vi "client example - sine wave - analog.vi"() -> ()   [LabVIEW 2021]
uses:
  controls/generation status.ctl
  controls/sine wave properties.ctl
  controls/analog output settings.ctl
  controls/terminal configuration.ctl
  AudioGeneration/Configure - Analog.vi
  AudioGeneration/AudioGeneration.lvclass
  controls/AudioGenTypeDefs.lvlib
panel:
  in  "sine wave properties":T1=[{"frequency"=1000.0, "amplitude"=1.0, "phase"=0.0}, {"frequency"=1000.0, "amplitude"=2.0, "phase"=30.0}]
  in  "update":bool
  in  "terminal configuration":i32(ring)=10106 items=["Default"=-1, "RSE"=10083, "Differential"=10106, "Pseudodifferential"=12529]
  in  "range":dbl=5.0
  in  "DAQmx Physical Channel":tag="PXI1Slot4/ao0:1"
  out "status":T2
  in  "stop":bool
  out "error out":errorcluster
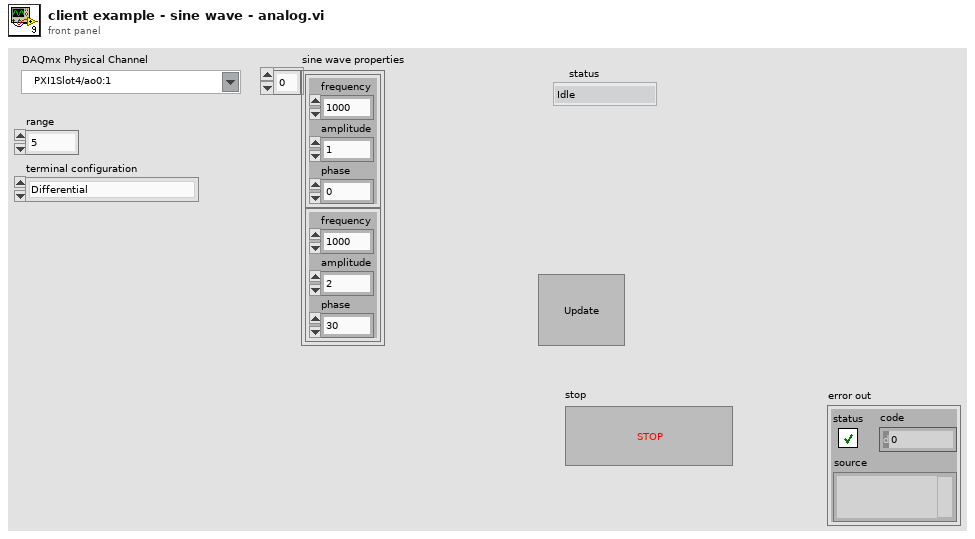
[diagram p1: front panel]
types:
  T1 = typedef "AudioGenTypeDefs.lvlib/sine wave properties.ctl" = cluster{"frequency":dbl, "amplitude":dbl, "phase":dbl}[]
  T2 = typedef "AudioGenTypeDefs.lvlib/generation status.ctl" = enum16{"Idle", "Committed", "Active"}
  T3 = typedef "AudioGenTypeDefs.lvlib/analog output settings.ctl" = cluster{"output rate":dbl, "range":dbl, "terminal configuration":T4, "output impedance":dbl, "common mode offset":dbl, "pure tone mode":bool}
  T4 = typedef "AudioGenTypeDefs.lvlib/terminal configuration.ctl" = enum32{"Default", "RSE", "Differential", "Pseudodifferential"}
  T5 = typedef "AudioGenTypeDefs.lvlib/signal settings.ctl" = cluster{"signal type":T6, "properties":string, "output level units":T7}
  T6 = typedef "AudioGenTypeDefs.lvlib/signal type.ctl" = enum16{"Sine", "Dual Tone"}
  T7 = typedef "audio controls.lvlib/digital output level units.ctl" = enum32{"% FS", "dBFS", "V"}
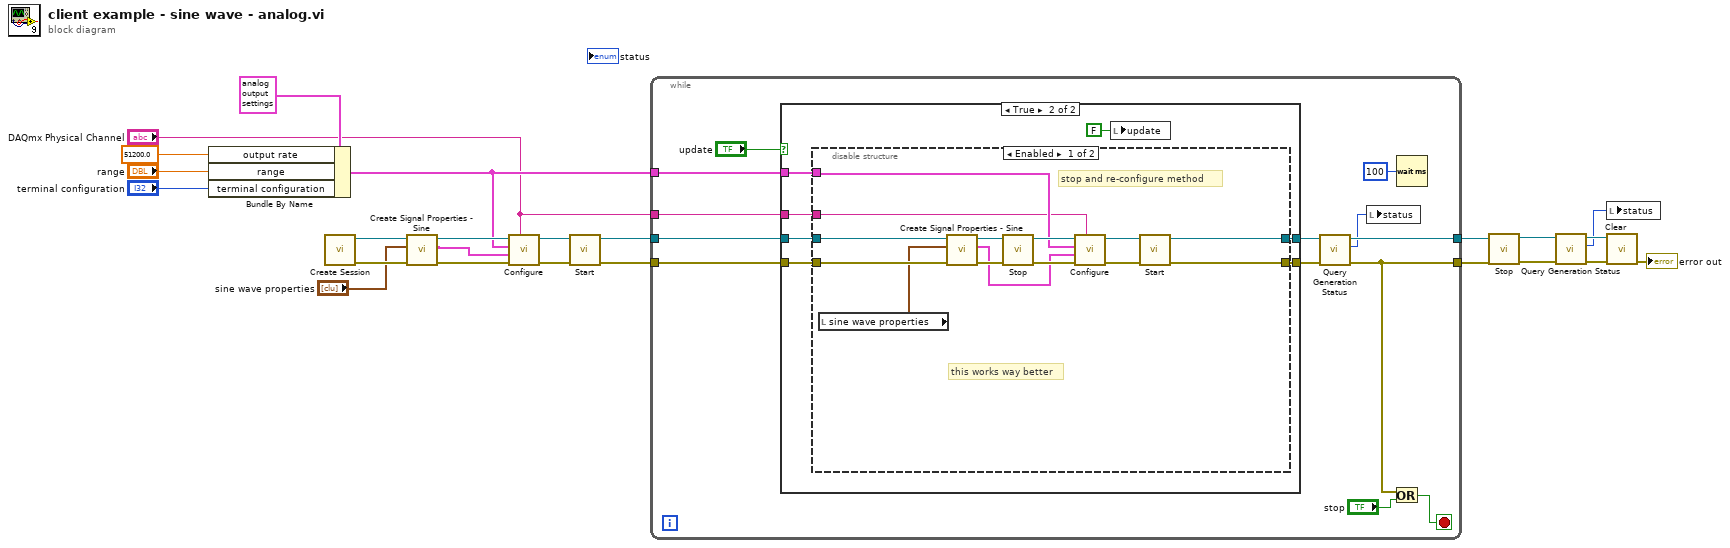
[diagram p0: block diagram]
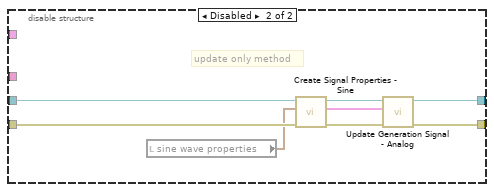
[diagram p3: hidden frame]
diagram:
  n1 = Bundle By Name(cluster=T3 {"output rate"=51200.0, "range"=5.0, "terminal configuration"=enum."Pseudodifferential", "output impedance"=0.0, "common mode offset"=0.0, "pure tone mode"=FALSE} ("output settings"), "output rate"=51200.0 ("output settings.output rate"), "range"="range", "terminal configuration"="terminal configuration") -> (w2:T3)
  n2 = call "Create Session.vi"() -> ("error out"=w9:errorcluster, "session out"=w10:refnum<class "AudioGeneration.lvclass">)  [unwired: 10 in]
  n3 = call "Create Signal Properties - Sine.vi"("error in (no error)"=w9, "sine wave properties"="sine wave properties", "AudioGeneration in"=w10) -> ("error out"=w6:errorcluster, "signal settings"=w7:T5, "AudioGeneration out"=w8:refnum<class "AudioGeneration.lvclass">)  [unwired: 6 in]
  n4 = call-poly "Configure.vi"("DAQmx Physical Channel"="DAQmx Physical Channel", "error in (no error)"=w6, "signal settings"=w7, "output settings"=w2, "AudioGeneration in"=w8) -> ("error out"=w4:errorcluster, "AudioGeneration out"=w5:refnum<class "AudioGeneration.lvclass">)  [unwired: 5 in]
  n5 = call "Start.vi"("error in (no error)"=w4, "AudioGeneration in"=w5) -> ("error out"=w20:errorcluster, "AudioGeneration out"=w21:refnum<class "AudioGeneration.lvclass">)  [unwired: 8 in]
  n6 = while {
    tunnel: [w34] -> w23
    tunnel: [w33] -> w22
    tunnel: w21 -> [w31]
    tunnel: w20 -> [w29]
    tunnel: w2 -> [w26]
    tunnel: "DAQmx Physical Channel" -> [w25]
    stop <- w36 stop-if-true
    n7 = case shown="True" "update" {
      tunnel: w31 -> [w39 w43]
      tunnel: w29 -> [w38 w42]
      tunnel: [w38 w46] -> w28
      tunnel: [w39 w45] -> w27
      tunnel: w26 -> [_ w41]
      tunnel: w25 -> [_ w40]
      frame False {
      }
      frame True {
        n8 = disable-structure shown="Enabled" {
          disable-tunnel: [w48 w68] -> w46
          disable-tunnel: [w49 w67] -> w45
          disable-tunnel: w43 -> [w60 w66]
          disable-tunnel: w42 -> [w59 w65]
          disable-tunnel: w41 -> [w53 _]
          disable-tunnel: w40 -> [w47 _]
          frame Enabled {
            # "this works way better"
            # "stop and re-configure method"
            n9 = local read "sine wave properties"() -> (w58:T1)
            n10 = call "Create Signal Properties - Sine.vi"("error in (no error)"=w59, "sine wave properties"=w58, "AudioGeneration in"=w60) -> ("error out"=w57:errorcluster, "signal settings"=w52:T5, "AudioGeneration out"=w56:refnum<class "AudioGeneration.lvclass">)  [unwired: 6 in]
            n11 = call "Stop.vi"("error in (no error)"=w57, "AudioGeneration in"=w56) -> ("error out"=w55:errorcluster, "AudioGeneration out"=w54:refnum<class "AudioGeneration.lvclass">)  [unwired: 8 in]
            n12 = call-poly "Configure.vi"("DAQmx Physical Channel"=w47, "error in (no error)"=w55, "signal settings"=w52, "output settings"=w53, "AudioGeneration in"=w54) -> ("error out"=w51:errorcluster, "AudioGeneration out"=w50:refnum<class "AudioGeneration.lvclass">)  [unwired: 5 in]
            n13 = call "Start.vi"("error in (no error)"=w51, "AudioGeneration in"=w50) -> ("error out"=w48:errorcluster, "AudioGeneration out"=w49:refnum<class "AudioGeneration.lvclass">)  [unwired: 8 in]
          }
          frame Disabled {
            # "update only method"
            n14 = local read "sine wave properties"() -> (w61:T1)
            n15 = call "Create Signal Properties - Sine.vi"("error in (no error)"=w65, "sine wave properties"=w61, "AudioGeneration in"=w66) -> ("error out"=w63:errorcluster, "signal settings"=w62:T5, "AudioGeneration out"=w64:refnum<class "AudioGeneration.lvclass">)  [unwired: 6 in]
            n16 = call "Update Generation Signal - Analog.vi"("error in (no error)"=w63, "signal settings"=w62, "AudioGeneration in"=w64) -> ("error out"=w68:errorcluster, "AudioGeneration out"=w67:refnum<class "AudioGeneration.lvclass">)  [unwired: 7 in]
          }
        }
        n17 = local write "update"(FALSE ("update")) -> ()
      }
    }
    n18 = call "Query Generation Status.vi"("error in (no error)"=w28, "AudioGeneration in"=w27) -> ("error out"=w33:errorcluster, "status"=w32:T2, "AudioGeneration out"=w34:refnum<class "AudioGeneration.lvclass">)  [unwired: 5 in, 2 out]
    n19 = local write "status"(w32) -> ()
    n20 = Or(x=w33, y="stop") -> (x .or. y?=w36:bool)
    n21 = Wait (ms)(milliseconds to wait=u32 100) -> ()  [unwired: 1 out]
  }
  n22 = call "Stop.vi"("error in (no error)"=w22, "AudioGeneration in"=w23) -> ("error out"=w15:errorcluster, "AudioGeneration out"=w19:refnum<class "AudioGeneration.lvclass">)  [unwired: 8 in]
  n23 = call "Query Generation Status.vi"("error in (no error)"=w15, "AudioGeneration in"=w19) -> ("error out"=w17:errorcluster, "status"=w16:T2, "AudioGeneration out"=w18:refnum<class "AudioGeneration.lvclass">)  [unwired: 5 in, 2 out]
  n24 = local write "status"(w16) -> ()
  n25 = call "Clear.vi"("error in (no error)"=w17, "AudioGeneration in"=w18) -> ("error out"=→"error out":errorcluster)  [unwired: 9 in]
